vi "get_config_cluster.vi"(8 "error in (no error)":errorcluster, 11 "TrajectoryAK101022Resonance in":refnum<class "TrajectoryAK101022Resonance.lvclass">) -> (0 "error out":errorcluster, 2 "config cluster (variant)":variant, 3 "TrajectoryAK101022Resonance out":refnum<class "TrajectoryAK101022Resonance.lvclass">)   [LabVIEW 2010, in "TrajectoryAK101022Resonance.lvclass"]
uses:
  TrajectoryAK101022Resonance.lvclass
  TrajectoryAK101022Resonance.lvclass/TrajectoryAK101022Resonance.ctl
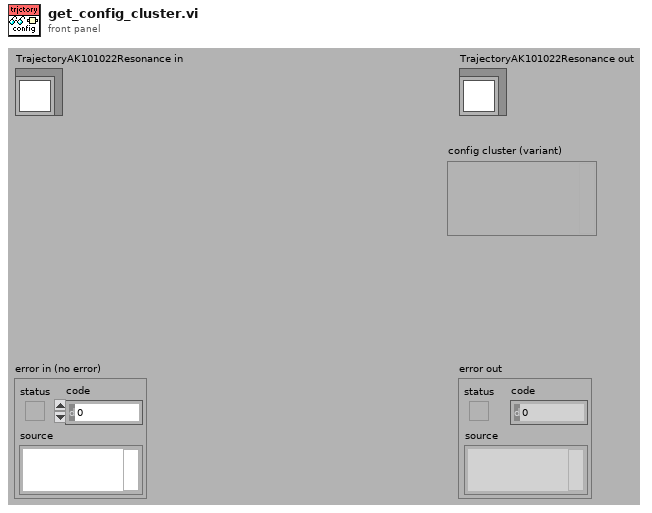
[diagram p1: front panel]
types:
  T1 = typedef "TrajectoryAK101022Resonance.lvclass/config_data_cluster.ctl" = cluster{"resonance frequency":dbl[unit], "no. of y-brake lines before flyback":i32, "no. of y-flyback lines":i32, "no. of y-brake lines after flyback":i32, "maximum x scanner value":dbl, "maximum y scanner value":dbl, "fly-forward offset default":dbl, "fly-back offset default":dbl, "scan segment default":dbl, "FOVx":dbl[unit], "FOVy":dbl[unit], "objective magnification":dbl, "component specification":T2, "number of y-fly-back steps":u16, "ETL current to Hifo-Box conversion":dbl[unit], "ETL current offset":dbl[unit]}
  T2 = typedef "plugin_specification.ctl" = cluster{"class path":string, "configuration":string, "label":string, "settings name":string}
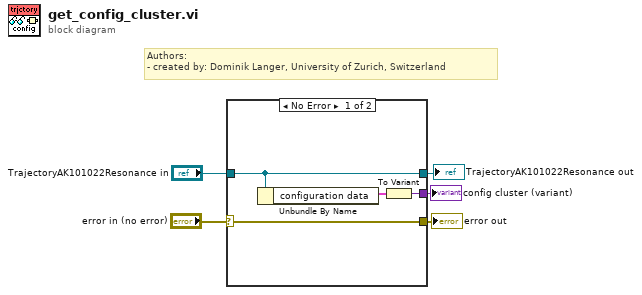
[diagram p0: block diagram]
diagram:
  # "Authors: \n- created by: Dominik Langer, University of Zurich, Switzerland"
  n1 = case shown="No Error" "error in (no error)" {
    selector: "error in (no error)" -> [w6 w10]
    tunnel: "TrajectoryAK101022Resonance in" -> [w7 w11]
    tunnel: [w9 _] -> w3
    tunnel: [w7 w11] -> w2
    tunnel: [w6 w10] -> w1
    frame No Error {
      n2 = Unbundle By Name(w7) -> ("configuration data"=w8:T1)
      n3 = To Variant(anything=w8) -> (Variant=w9:variant)
    }
    frame Error {
    }
  }
  "error out" <- w1
  "TrajectoryAK101022Resonance out" <- w2
  "config cluster (variant)" <- w3
